vi "test_yaqc_measure.vi"() -> ()   [LabVIEW 2022 SP3]
uses:
  1804933d-d101-43a8-95ba-f569bdd17e4f.vi
  c345092d-4fa4-4084-98a0-1db564c1fa05.vi
  yaq_labview/yaq_labview_error_handler.vi
  <vilib>/Utility/error.llb/Simple Error Handler.vi
panel:
  out "USB2000":cluster{"X Array Out":dbl[], dbl[]}(graph)
  in  "Port":i32=39004
  in  "Stop":bool
  in  "Python Module Path":path
  in  "Python version":string="3.8.0"
  in  "Python path":path=path "C:/ProgramData/Anaconda3/envs/lv4/pythonw.exe"
  # "C:\\ProgramData\\Anaconda3\\envs\\XXXXXX\\python.exe  for Anaconda pkgs"
  # "Path to yaqc_labview.py, which may be located in LabVIEW 2022's instr.lib folder."
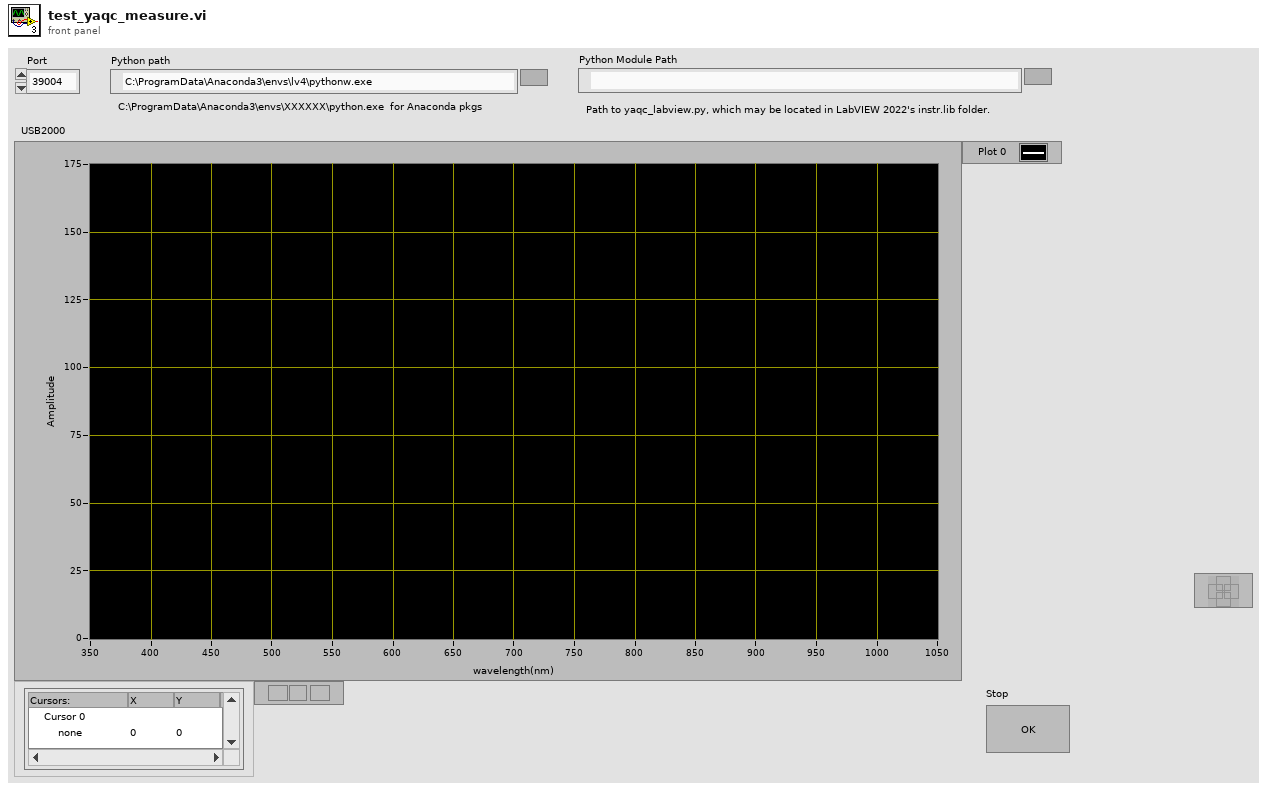
[diagram p1: front panel]
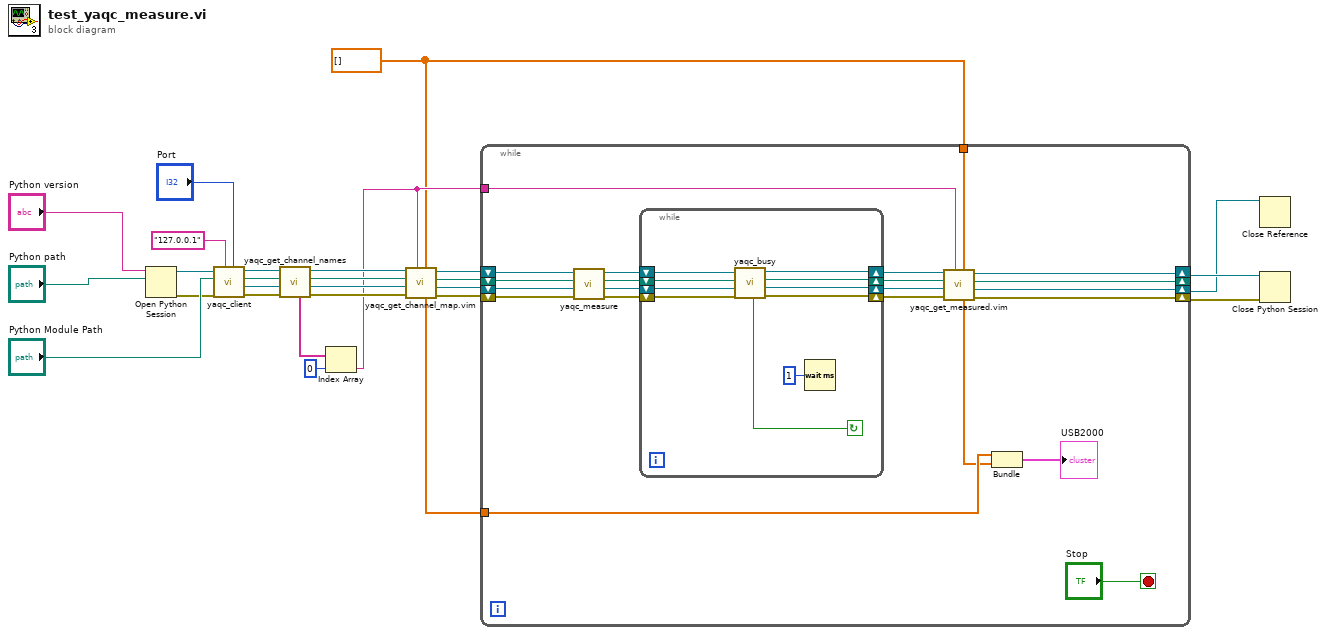
[diagram p0: block diagram]
diagram:
  w5 = dbl[] []
  n1 = Open Python Session(python version="Python version", python path="Python path") -> (session out=w2:refnum<k35>, error out=w1:errorcluster)  [unwired: 1 in]
  n2 = call "yaqc_client.vi"("Port"="Port", "host ('127.0.0.1')"="127.0.0.1", "error in (no error)"=w1, "Python Module Path"="Python Module Path", "Python Session In"=w2) -> ("error out"=w14:errorcluster, "Yaqc Client"=w12:refnum<k38>, "Python Module Path Out"=w3:path, "Python Session Out"=w4:refnum<k35>)  [unwired: 3 in]
  n3 = call "yaqc_get_channel_names.vi"("error in (no error)"=w14, "Yaqc Client In"=w12, "Python Module Path In"=w3, "Python Session In"=w4) -> ("error out"=w13:errorcluster, "Yaqc Client Out"=w11:refnum<k38>, "Python Module Path Out"=w10:path, "Python Session Out"=w9:refnum<k35>, "Channel Names Out"=w8:string[])  [unwired: 3 in]
  n4 = Index Array(array=w8, index=0) -> (element=w6:string)
  n5 = call "yaqc_get_channel_map.vim"("Map In"=w5, "channel_name"=w6, "error in (no error)"=w13, "Yaqc Client In"=w11, "Python Module Path In"=w10, "Python Session In"=w9) -> ("error out"=w19:errorcluster, "Yaqc Client Out"=w18:refnum<k38>, "Python Module Path Out"=w17:path, "Python Session Out"=w16:refnum<k35>, "Map Out"=w15:dbl[])  [unwired: 1 in]
  n6 = while {
    shift-right: [w45] -> w24
    shift-left: w19 -> [w46]
    shift-right: [w44] -> w22
    shift-left: w18 -> [w47]
    shift-right: [w43] -> _
    shift-left: w17 -> [w48]
    shift-right: [w42] -> w23
    shift-left: w16 -> [w49]
    tunnel: w15 -> [w40]
    tunnel: w5 -> [w39]
    tunnel: w6 -> [w38]
    stop <- "Stop" stop-if-true
    n7 = call "yaqc_measure.vi"("error in (no error)"=w46, "Yaqc Client In"=w47, "Python Module Path In"=w48, "Python Session In"=w49) -> ("error out"=w34:errorcluster, "Yaqc Client Out"=w35:refnum<k38>, "Python Module Path Out"=w36:path, "Python Session Out"=w37:refnum<k35>)  [unwired: 4 in]
    n8 = while {
      shift-right: [w55] -> w32
      shift-left: w34 -> [w59]
      shift-right: [w54] -> w31
      shift-left: w35 -> [w58]
      shift-right: [w53] -> w30
      shift-left: w36 -> [w57]
      shift-right: [w52] -> w29
      shift-left: w37 -> [w56]
      stop <- w51 continue-if-true
      n9 = call "yaqc_busy.vi"("error in (no error)"=w59, "Yaqc Client In"=w58, "Python Module Path In"=w57, "Python Session In"=w56) -> ("error out"=w55:errorcluster, "Yaqc Client Out"=w54:refnum<k38>, "Python Module Path Out"=w53:path, "Python Session Out"=w52:refnum<k35>, "busy?"=w51:bool)  [unwired: 3 in]
      n10 = Wait (ms)(milliseconds to wait=u32 1) -> ()  [unwired: 1 out]
    }
    n11 = call "yaqc_get_measured.vim"("Measured In"=w39, "Channel_name"=w38, "error in (no error)"=w32, "Yaqc Client In"=w31, "Python Module Path In"=w30, "Python Session In"=w29) -> ("error out"=w45:errorcluster, "Yaqc Client Out"=w44:refnum<k38>, "Python Module Path Out"=w43:path, "Python Session Out"=w42:refnum<k35>, "Measured Out"=w28:dbl[])  [unwired: 1 in]
    n12 = Bundle("Map Out"=w40, "Measured Out"=w28) -> (→"USB2000":cluster{"Map Out":dbl[], "Measured Out":dbl[]})  [unwired: 1 in]
  }
  n13 = Close Reference(reference=w22) -> ()  [unwired: 1 in, 1 out]
  n14 = Close Python Session(session in=w23, error in=w24) -> ()  [unwired: 1 out]
